vi "ADO Recordset Create.vi"(8 "error in (no error)":errorcluster) -> (0 "error out":errorcluster, 3 "ADODB._Recordset Out":refnum<k7>)   [LabVIEW 2013]
panel:
  in  "ADODB._Recordset":refnum<k7>
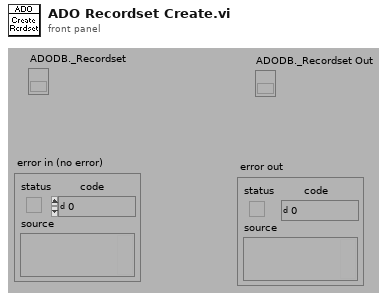
[diagram p1: front panel]
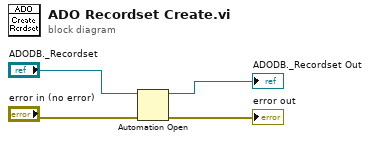
[diagram p0: block diagram]
diagram:
  n1 = Automation Open(error in (no error)="error in (no error)", Automation Refnum="ADODB._Recordset") -> (Automation Refnum=→"ADODB._Recordset Out":refnum<k7>, error out=→"error out":errorcluster)  [unwired: 2 in]
